vi "SetCurrentGain.vi"(3 "Gain":enum16{"1", "2", "3", "4"}(ring), 4 "Device":u8=1, 5 "Serial port":refnum<visa-resource-name>) -> (1 "Device out":u8=1, 2 "Serial port out":refnum<visa-resource-name>)   [LabVIEW 2021]
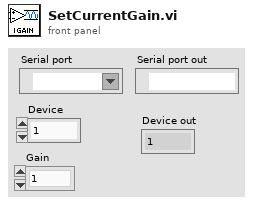
[diagram p1: front panel]
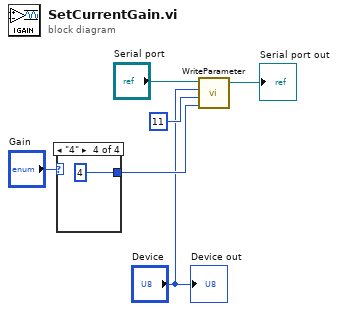
[diagram p0: block diagram]
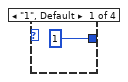
[diagram p2: hidden frame]
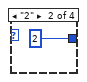
[diagram p3: hidden frame]
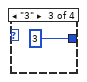
[diagram p4: hidden frame]
diagram:
  n1 = case shown="\"4\"" "Gain" {
    tunnel: [1 2 3 4] -> w2
    frame "1", Default {
    }
    frame "2" {
    }
    frame "3" {
    }
    frame "4" {
    }
  }
  n2 = call "WriteParameter.vi"("Value"=w2, "Address"=u32 11, "Device"="Device", "Serial port"="Serial port") -> ("Serial port out"=→"Serial port out":refnum<visa-resource-name>)  [unwired: 2 in]
  "Device out" <- "Device"
